vi "cw_4_2.vi"() -> ()   [LabVIEW 2022 SP3]
uses:
  <vilib>/numeric/Random Number (Range) U64.vi
  <vilib>/numeric/sub_Random U32.vi
panel:
  in  "stop":bool
  out "Array":i32[](array[numeric])
  in  "Boolean":bool
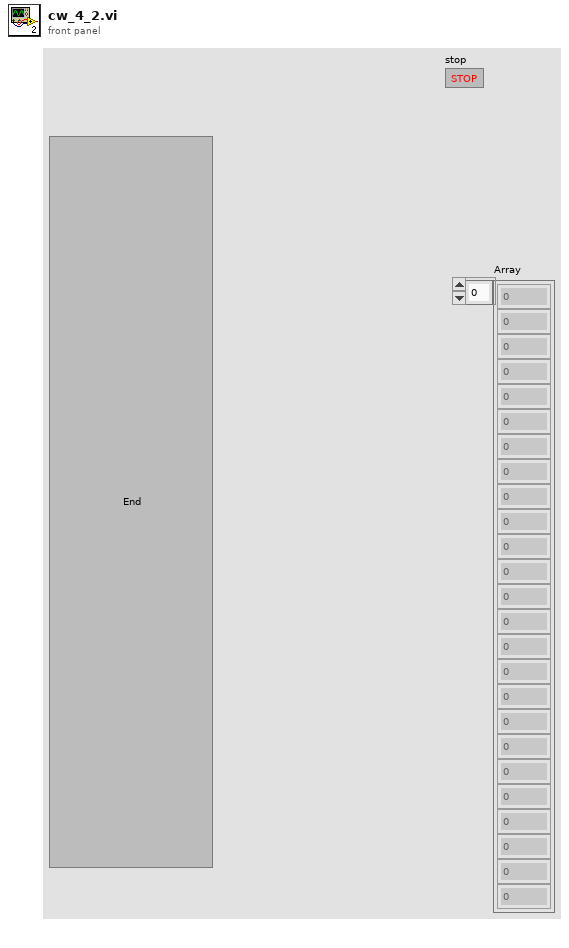
[diagram p1: front panel]
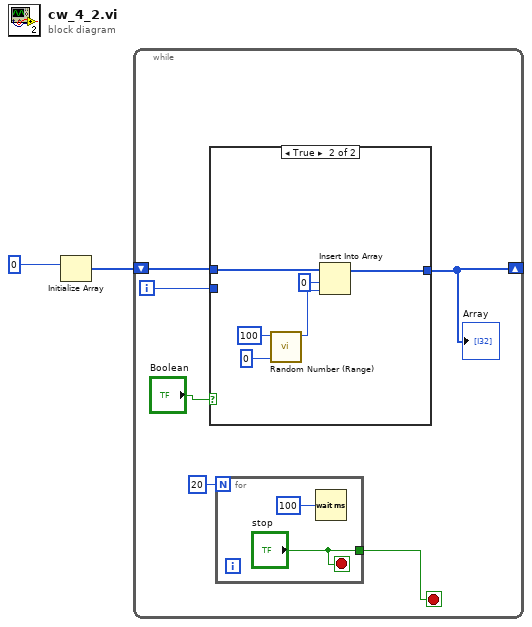
[diagram p0: block diagram]
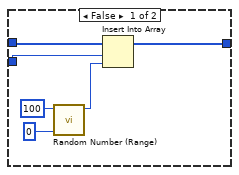
[diagram p2: hidden frame]
diagram:
  n1 = Initialize Array(0 ("element")) -> (w2:i32[])  [unwired: 1 in]
  n2 = while {
    shift-right: [w5] -> _
    shift-left: w2 -> [w6]
    i -> [w7]
    stop <- w4 stop-if-true
    n3 = case shown="True" "Boolean" {
      tunnel: w7 -> [w12 _]
      tunnel: w6 -> [w13 w19]
      tunnel: [w11 w18] -> w5
      frame False {
        n4 = call-poly <vilib>:"Random Number (Range).vi"("lower bound (0)"=u64 0, "upper bound (100)"=u64 100) -> ("number"=w16:u64)  [unwired: 9 in]
        n5 = Insert Into Array(array=w13, index=w12, new element=w16) -> (w11:i32[])
      }
      frame True {
        n6 = call-poly <vilib>:"Random Number (Range).vi"("lower bound (0)"=u64 0, "upper bound (100)"=u64 100) -> ("number"=w22:u64)  [unwired: 9 in]
        n7 = Insert Into Array(array=w19, index=0, new element=w22) -> (w18:i32[])
      }
    }
    "Array" <- w5
    n8 = for {
      N: 20 -> [_]
      tunnel: ["stop"] -> w4
      stop <- "stop" stop-if-true
      n9 = Wait (ms)(milliseconds to wait=u32 100) -> ()  [unwired: 1 out]
    }
  }
